vi "Generator.Create AO waveforms.vi"(8 "error in (no error)":errorcluster, 10 "reset phase":bool, 11 "Lockin.DAQ":refnum<class "Instrument.DAQ.lvclass">) -> (0 "error out":errorcluster, 2 "AO Array":waveform(dbl)[](array[waveform]), 3 "Lockin.DAQ out":refnum<class "Instrument.DAQ.lvclass">)   [LabVIEW 2019, in "Instrument.Lockin.lvlib" / "Instrument.DAQ.lvclass"]
uses:
  Instrument.DAQ.lvclass
  Typedefs/AO.Channel--Cluster--Array.ctl
  Typedefs/AO.Channel--Cluster.ctl
  Typedefs/AO.Channel.Function--Enum.ctl
  Instrument.DAQ.lvclass/Instrument.DAQ.ctl
  <vilib>/Waveform/WDTOps.llb/WDT Append Waveforms DBL.vi
  <vilib>/measure/NI_MABase.lvlib
  Typedefs/DAQ.Sampling.Sampling--Cluster.ctl
panel:
  in  "Tab Control":enum32{"Page 1", "Graphs"}(tab)
  in  "Channels: AO":T1 {"Phase" format="%.3g"; "Frequency" min=0.0001 max=10000.0 format="%.3g"; "Offset" format="%.3p"; "Amplitude" min=0.0 max=10.0 format="%.3p"}
  in  "y":dbl format="%#_13g"
  out "Waveform Graph":waveform(dbl)[](graph)
  out "Waveform Chart":dbl[][](graph)
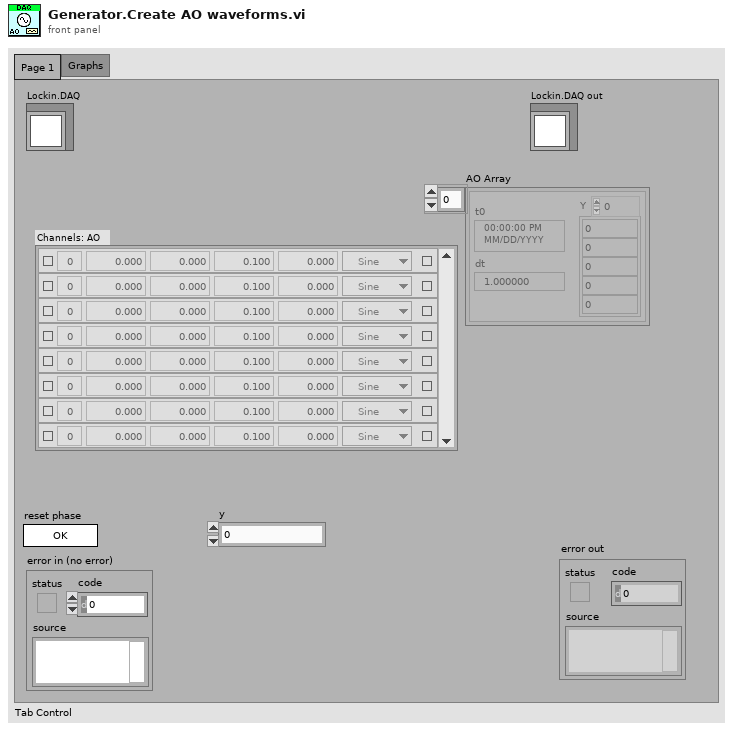
[diagram p1: front panel]
types:
  T1 = typedef "Instrument.Lockin.lvlib/Instrument.DAQ.lvclass/AO.Channel--Cluster--Array.ctl" = T2[]
  T2 = typedef "Instrument.Lockin.lvlib/Instrument.DAQ.lvclass/AO.Channel--Cluster.ctl" = cluster{"Enable?":bool, "Channel":i32, "Amplitude":dbl, "Offset":dbl, "Frequency":dbl, "Phase":dbl, "Function":T3, "Sweeping?":bool}
  T3 = typedef "Instrument.Lockin.lvlib/Instrument.DAQ.lvclass/AO.Channel.Function--Enum.ctl" = enum16{"Sine", "Triangle", "Square"}
  T4 = typedef "Instrument.Lockin.lvlib/Instrument.DAQ.lvclass/REF.Channel--Cluster--Array.ctl" = T5[]
  T5 = typedef "Instrument.Lockin.lvlib/Instrument.DAQ.lvclass/REF.Channel--Cluster.ctl" = cluster{"Enable?":bool, "Channel":i32, "Frequency":dbl, "Phase":dbl, "TC":dbl, "Roll-Off":i32}
  T6 = typedef "Instrument.Lockin.lvlib/Instrument.DAQ.lvclass/DAQ.Sampling.Sampling--Cluster.ctl" = cluster{"Fs":dbl, "#s":i32}
  T7 = enum16{"Sine Wave", "Triangle Wave", "Square Wave", "Sawtooth Wave"}
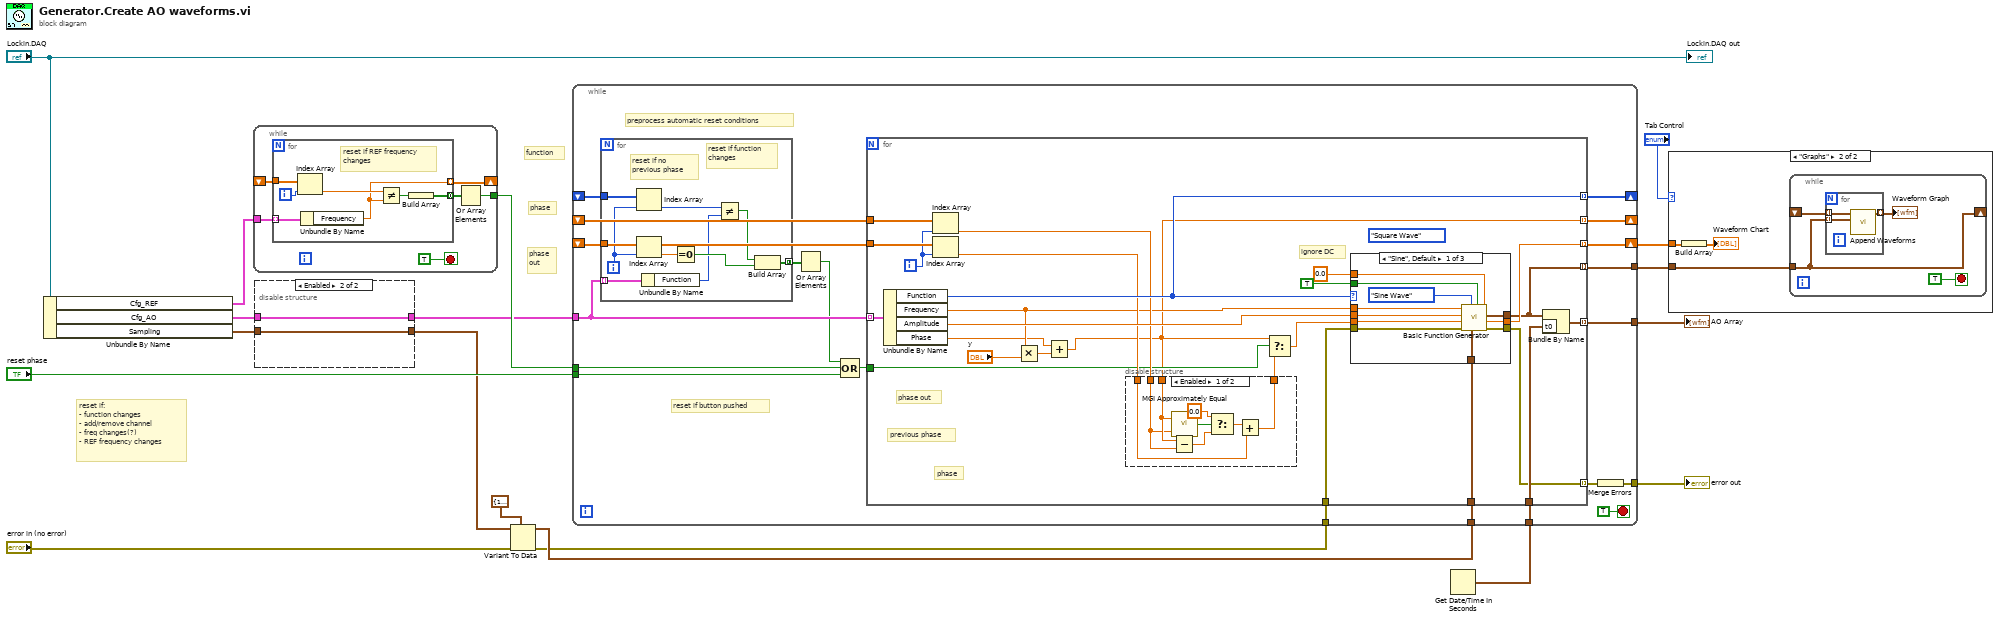
[diagram p0: block diagram]
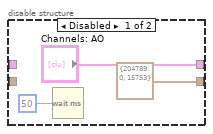
[diagram p2: hidden frame]
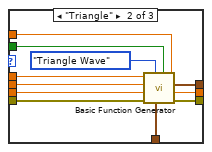
[diagram p4: hidden frame]
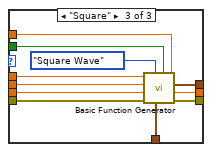
[diagram p5: hidden frame]
diagram:
  # "phase"
  # "function"
  # "phase\nout"
  # "reset if:\n- function changes\n- add/remove channel\n- freq changes(?)\n- REF frequency changes"
  n1 = Unbundle By Name("Lockin.DAQ") -> ("Cfg_REF"=w9:T4, "Cfg_AO"=w13:T1, "Sampling"=w12:T6)
  n2 = while {
    tunnel: w9 -> [w24]
    shift-right: [w23] -> _
    shift-left: _ -> [w22]
    tunnel: [w19] -> w10
    stop <- TRUE stop-if-true
    n3 = for {
      tunnel: w24 -> [w26] mode=indexing
      tunnel: w22 -> [w30]
      tunnel: [w27] -> w20 mode=concatenating
      tunnel: [w25] -> w23 mode=indexing
      i -> [w31]
      # "reset if REF frequency\nchanges"
      n4 = Index Array(array=w30, index=w31) -> (element=w29:dbl)
      n5 = Unbundle By Name(w26) -> ("Frequency"=w25:dbl)
      n6 = Not Equal?(x=w29, y=w25) -> (x != y?=w28:bool)
      n7 = Build Array(w28) -> (w27:bool[])
    }
    n8 = Or Array Elements(Boolean array=w20) -> (logical OR=w19:bool)
  }
  n9 = disable-structure shown="Enabled" {
    disable-tunnel: [T6 {"Fs"=204789.0, "#s"=15753} ("Configuration.DAQ.sampling") w35] -> w1
    disable-tunnel: w13 -> [_ w36]
    disable-tunnel: w12 -> [_ w35]
    disable-tunnel: ["Channels: AO" w36] -> w7
    frame Disabled {
      n10 = Wait (ms)(milliseconds to wait=u32 50) -> ()  [unwired: 1 out]
    }
    frame Enabled {
    }
  }
  n11 = Variant To Data(error in="error in (no error)", type=cluster{"Fs":dbl, "#s":dbl} {"Fs"=1000.0, "#s"=1000.0} ("sampling info"), Variant=w1) -> (data=w4:cluster{"Fs":dbl, "#s":dbl}, error out=w2:errorcluster)
  n12 = Get Date/Time In Seconds() -> (seconds since 1Jan1904=w17:timestamp)
  n13 = while {
    tunnel: w4 -> [w56]
    tunnel: [w55] -> w14
    shift-right: [w53] -> w11
    shift-left: _ -> [w42]
    tunnel: w17 -> [w52]
    tunnel: "reset phase" -> [w46]
    tunnel: w2 -> [w51]
    tunnel: [w49] -> w16
    tunnel: w7 -> [w48]
    shift-right: [w44] -> _
    shift-left: _ -> [w43]
    shift-right: [w41] -> _
    shift-left: _ -> [w40]
    tunnel: w10 -> [w39]
    tunnel: [w38] -> w8
    stop <- TRUE stop-if-true
    # "reset if button pushed"
    # "preprocess automatic reset conditions"
    n14 = for {
      tunnel: w48 -> [w58] mode=indexing
      tunnel: w42 -> [w65]
      tunnel: w43 -> [w64]
      tunnel: [w59] -> w47 mode=concatenating
      i -> [w66]
      # "reset if function\nchanges"
      # "reset if no\nprevious phase"
      n15 = Index Array(array=w64, index=w66) -> (element=w62:T3)
      n16 = Index Array(array=w65, index=w66) -> (element=w63:dbl)
      n17 = Unbundle By Name(w58) -> ("Function"=w57:T3)
      n18 = Equal To 0?(x=w63) -> (x = 0?=w60:bool)
      n19 = Not Equal?(x=w62, y=w57) -> (x != y?=w61:bool)
      n20 = Build Array(w61, w60) -> (w59:bool[])
    }
    n21 = Or Array Elements(Boolean array=w47) -> (logical OR=w37:bool)
    n22 = Compound Arithmetic op=OR(w37, w39, w46) -> (w45:bool)
    n23 = for {
      tunnel: [w89] -> w55 mode=indexing
      tunnel: w56 -> [w87]
      tunnel: [w73] -> w53 mode=indexing
      tunnel: w52 -> [w91]
      tunnel: w51 -> [w85]
      tunnel: [w88] -> w50 mode=indexing
      tunnel: w48 -> [w84] mode=indexing
      tunnel: w45 -> [w74]
      tunnel: [w82] -> w44 mode=indexing
      tunnel: w42 -> [w81]
      tunnel: [w67] -> w41 mode=indexing
      tunnel: w40 -> [w77]
      tunnel: [w72] -> w38 mode=indexing
      i -> [w80]
      (unwired) T7."Square Wave" ("signal type")
      # "previous phase"
      # "phase"
      # "phase out"
      # "ignore DC"
      n24 = Unbundle By Name(w84) -> ("Function"=w82:T3, "Frequency"=w69:dbl, "Amplitude"=w83:dbl, "Phase"=w68:dbl)
      n25 = Index Array(array=w77, index=w80) -> (element=w78:dbl)
      n26 = Index Array(array=w81, index=w80) -> (element=w79:dbl)
      n27 = Multiply(x=w69, y="y") -> (x*y=w70:dbl)
      n28 = Add(x=w68, y=w70) -> (x+y=w67:dbl)
      n29 = disable-structure shown="Enabled" {
        disable-tunnel: w67 -> [w98 _]
        disable-tunnel: w78 -> [w97 _]
        disable-tunnel: w79 -> [w92 w100]
        disable-tunnel: [w95 w100] -> w76
        frame Enabled {
          n30 = call <userlib>:"MGI Approximately Equal.vi"("Numeric 2"=w97, "Numeric 1"=w98) -> ("approx = ?"=w96:bool)
          n31 = Subtract(x=w98, y=w97) -> (x-y=w94:dbl)
          n32 = Select(t=0.0, s=w96, f=w94) -> (s? t:f=w93:dbl)
          n33 = Add(x=w93, y=w92) -> (x+y=w95:dbl)
        }
        frame Disabled {
        }
      }
      n34 = Select(t=w67, s=w74, f=w76) -> (s? t:f=w75:dbl)
      n35 = case shown="\"Sine\", Default" w82 {
        tunnel: w69 -> [w111 w122 w133]
        tunnel: 0.0 ("AO DC") -> [w110 w121 w132]
        tunnel: [w109 w120 w131] -> w72
        tunnel: TRUE ("reset signal") -> [w101 w112 w123]
        tunnel: w85 -> [w108 w119 w130]
        tunnel: [w107 w118 w129] -> w88
        tunnel: [w106 w117 w128] -> w73
        tunnel: w83 -> [w105 w116 w127]
        tunnel: w75 -> [w104 w115 w126]
        tunnel: w87 -> [w103 w114 w125]
        frame "Sine", Default {
          n36 = call <vilib>:"Basic Function Generator.vi"("offset"=w110, "reset signal"=w101, "sampling info"=w103, "signal type"=T7."Sine Wave", "error in (no error)"=w108, "phase"=w104, "amplitude"=w105, "frequency"=w111) -> ("error out"=w107:errorcluster, "phase out"=w106:dbl, "signal out"=w109:waveform(dbl))  [unwired: 1 in]
        }
        frame "Triangle" {
          n37 = call <vilib>:"Basic Function Generator.vi"("offset"=w121, "reset signal"=w112, "sampling info"=w114, "signal type"=T7."Triangle Wave", "error in (no error)"=w119, "phase"=w115, "amplitude"=w116, "frequency"=w122) -> ("error out"=w118:errorcluster, "phase out"=w117:dbl, "signal out"=w120:waveform(dbl))  [unwired: 1 in]
        }
        frame "Square" {
          n38 = call <vilib>:"Basic Function Generator.vi"("offset"=w132, "reset signal"=w123, "sampling info"=w125, "signal type"=T7."Square Wave", "error in (no error)"=w130, "phase"=w126, "amplitude"=w127, "frequency"=w133) -> ("error out"=w129:errorcluster, "phase out"=w128:dbl, "signal out"=w131:waveform(dbl))  [unwired: 1 in]
        }
      }
      n39 = Bundle By Name(cluster=w72, "t0"=w91) -> (w89:waveform(dbl))
    }
    n40 = Merge Errors(w50) -> (w49:errorcluster)
  }
  "AO Array" <- w14
  "error out" <- w16
  n41 = case shown="\"Graphs\"" "Tab Control" {
    tunnel: w8 -> [_ w134]
    tunnel: w11 -> [_ w135]
    frame Default {
    }
    frame "Graphs" {
      n42 = Build Array(w135) -> (→"Waveform Chart":dbl[][])
      n43 = while {
        shift-right: [w137] -> _
        shift-left: _ -> [w138]
        tunnel: w134 -> [w137]
        stop <- TRUE stop-if-true
        n44 = for {
          tunnel: [w143] -> w139 mode=indexing
          tunnel: w138 -> [w142] mode=indexing
          tunnel: w137 -> [w141] mode=indexing
          n45 = call-poly <vilib>:"Append Waveforms.vi"("waveform B"=w141, "waveform A"=w142) -> ("waveform out"=w143:waveform(dbl))  [unwired: 8 in, 1 out]
        }
        "Waveform Graph" <- w139
      }
    }
  }
  "Lockin.DAQ out" <- "Lockin.DAQ"
